vi "run.vi"(8 "error in (no error)":errorcluster, 11 "dotnet_system_exec in":refnum<class "dotnet_system_exec.lvclass">) -> (0 "error out":errorcluster, 3 "dotnet_system_exec out":refnum<class "dotnet_system_exec.lvclass">)   [LabVIEW 2020, in "dotnet_system_exec.lvclass"]
doc: "Runs the .NET System Process as configured with the @create method"
uses:
  dotnet_system_exec.lvclass
  dotnet_system_exec.lvclass/dotnet_system_exec.ctl
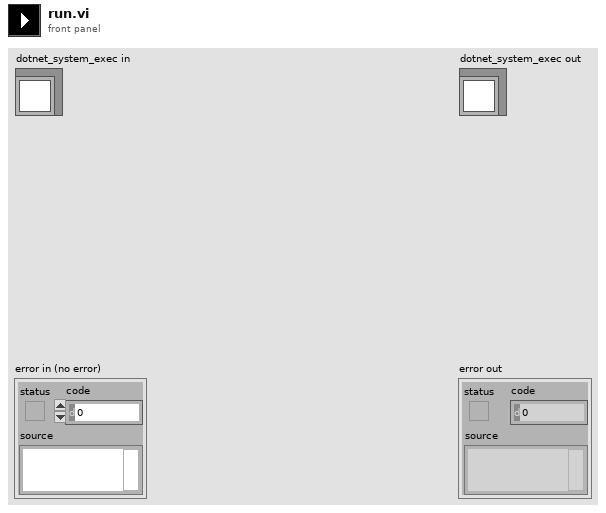
[diagram p1: front panel]
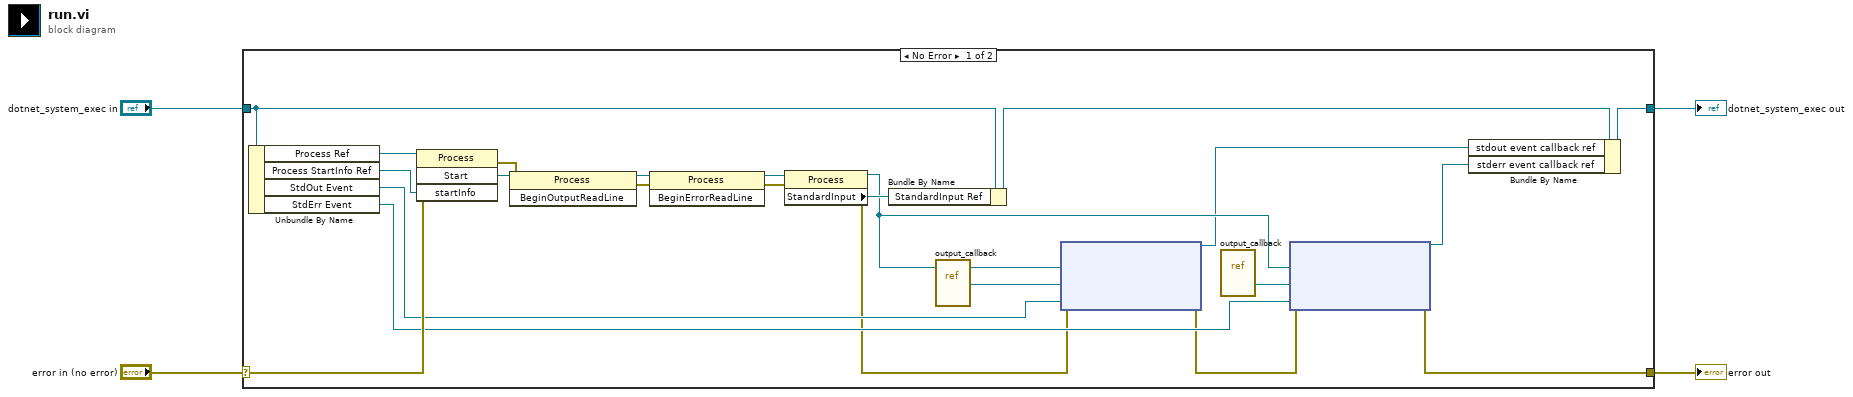
[diagram p0: block diagram]
diagram:
  n1 = case shown="No Error" "error in (no error)" {
    selector: "error in (no error)" -> [w19 w29]
    tunnel: [w12 w29] -> w3
    tunnel: [w9 w28] -> w1
    tunnel: "dotnet_system_exec in" -> [w18 w28]
    frame No Error {
      n2 = Unbundle By Name(w18) -> ("Process Ref"=w25:refnum<k24>, "Process StartInfo Ref"=w24:refnum<k24>, "StdOut Event"=w16:refnum<user-event>, "StdErr Event"=w15:refnum<user-event>)
      n3 = invoke class="Process" method="Start"(reference=w25, error in=w19, "startInfo"=w24) -> (error out=w23:errorcluster, "Start"=w22:refnum<k24>)  [unwired: 1 in, 2 out]
      n4 = invoke class="Process" method="BeginOutputReadLine"(reference=w22, error in=w23) -> (reference out=w27:refnum<k24>, error out=w26:errorcluster)  [unwired: 1 in, 1 out]
      n5 = invoke class="Process" method="BeginErrorReadLine"(reference=w27, error in=w26) -> (reference out=w21:refnum<k24>, error out=w20:errorcluster)  [unwired: 1 in, 1 out]
      n6 = property class="Process"(reference=w21, error in=w20) -> (reference out=w11:refnum<k24>, error out=w14:errorcluster, "StandardInput"=w17:refnum<k24>)
      n7 = Bundle By Name(cluster=w18, "StandardInput Ref"=w17) -> (w10:refnum<class "dotnet_system_exec.lvclass">)
      n8 = vi-ref "output_callback.vi"() -> ("vi reference"=w6:refnum<vi>)
      n9 = node(w14, w11, w6, w16) -> (w8:refnum<k27>, w13:errorcluster)  [unwired: 1 in]
      n10 = vi-ref "output_callback.vi"() -> ("vi reference"=w5:refnum<vi>)
      n11 = node(w13, w11, w5, w15) -> (w7:refnum<k27>, w12:errorcluster)  [unwired: 1 in]
      n12 = Bundle By Name(cluster=w10, "stdout event callback ref"=w8, "stderr event callback ref"=w7) -> (w9:refnum<class "dotnet_system_exec.lvclass">)
    }
    frame Error {
    }
  }
  "error out" <- w3
  "dotnet_system_exec out" <- w1
